vi "pi.calculate_backward_euler.vi"(6 "sampling_time (s)":dbl, 10 "Ti":dbl, 11 "Kc":dbl) -> (2 "a1...an":dbl[](array[numeric]), 3 "b0...bn":dbl[](array[numeric]))   [LabVIEW 2015, in "discrete_control_systems.lvlib"]
doc: "Calculates the gains for a discrete difference equation from the PI controller parameters using the backward euler discretization method.\n\nThe implemented controller has the following equation in the LaPlace domain, where U(s) is the controller output:\n\nU(s) = Kc * ( 1 + 1/(Ti*s) )"
uses:
  discrete_control_systems.lvlib
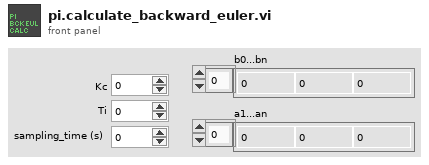
[diagram p1: front panel]
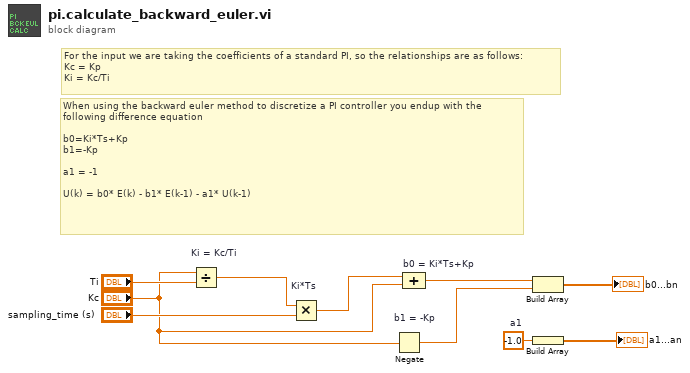
[diagram p0: block diagram]
diagram:
  w7 = -1.0  # a1
  # "For the input we are taking the coefficients of a standard PI, so the relationships are as follows:\nKc = Kp\nKi = Kc/Ti"
  # "When using the backward euler method to discretize a PI controller you endup with the\nfollowing difference equation\n\nb0=Ki*Ts+Kp\nb1=-Kp\n\na1 = -1\n\nU(k) = b0* E(k) - b1* E(k-1) - a1* U(k-1)"
  n1 = Divide "Ki = Kc/Ti"(x="Kc", y="Ti") -> (x/y=w9:dbl)
  n2 = Multiply "Ki*Ts"(x=w9, y="sampling_time (s)") -> (x*y=w8:dbl)
  n3 = Negate "b1 = -Kp"(x="Kc") -> (-x=w4:dbl)
  n4 = Compound Arithmetic op=ADD "b0 = Ki*Ts+Kp"(w8, "Kc") -> (w3:dbl)
  n5 = Build Array(w3, w4) -> (→"b0...bn":dbl[])
  n6 = Build Array(w7) -> (→"a1...an":dbl[])
